vi "Get Register.vi"(11 "Attributes in":refnum<class "Attributes.lvclass">) -> (2 "Register":refnum<event-registration>)   [LabVIEW 2020, in "jettl.lvlib" / "Attributes.lvlib" / "Attributes.lvclass"]
uses:
  Attributes.lvclass
  Msg/Msg.lvclass
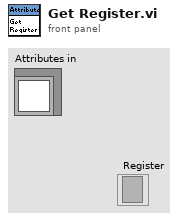
[diagram p1: front panel]
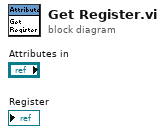
[diagram p0: block diagram]
diagram:
